vi "Circus Kaslis IPs.vi"(3 "error in (no error)":errorcluster, 4 "ID":string) -> (0 "error out":errorcluster, 1 "IP":string)   [LabVIEW 2026, in "TALOS.lvlib"]
doc: "This VI gives the IP of a PC, given its name, if it has been correctly inserted in the AEgIS_Config_Param.ini. If not present, it returns its ID (which is also its DNS name)."
uses:
  TALOS.lvlib
  Ancestor/Ancestor/Ancestor.lvclass/Ancestor.ctl
  FGV/Error Memory/Get Error Description.vi
  Get PC name.vi
  Ancestor/Ancestor/Read ID.vi
  Get Class Name.vi
  <vilib>/Utility/error.llb/Clear Errors.vi
  FGV/Error Memory/Error Memory Core.vi
  <vilib>/AdvancedString/Delimited String to 1D String Array (string).vi
  Circus Root Path.vi
  FGV/Error Memory/Error Crt Lvl checker.vi
  FGV/Error Memory/Error Memory Core.vi/40c8088d-b597-4017-91af-faa98e00292e.vi
  FGV/Error Memory/Error Memory Core.vi/d4a3ab98-063c-4e44-b43d-fbdcfe6c2be2.vi
  Global Memory.vi
  <vilib>/Utility/LVClass/Get LV Class Name.vi
  Is in Packed Library.vi
  TALOS Root path.vi
  Read CSV worksheet.vi
  Global Constants.vi
  <vilib>/Utility/error.llb/General Error Handler.vi
  Ancestor/Ancestor/Ancestor.lvclass
  <vilib>/Comparison/Equal/Equal Functor/Equal Functor.lvclass
  <vilib>/Utility/error.llb/Trim Whitespace (string).vi
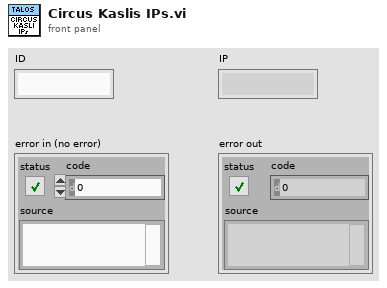
[diagram p1: front panel]
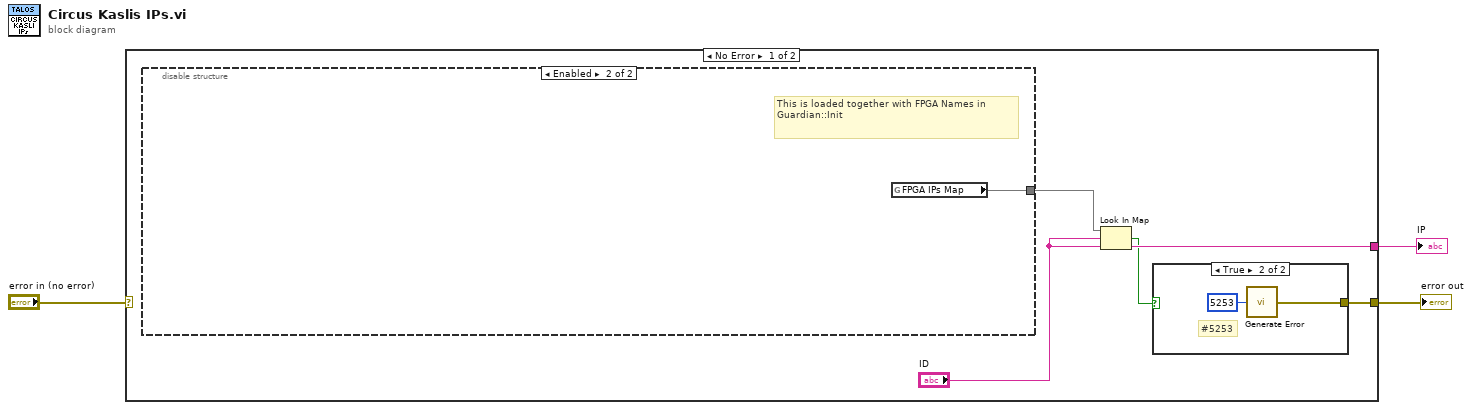
[diagram p0: block diagram]
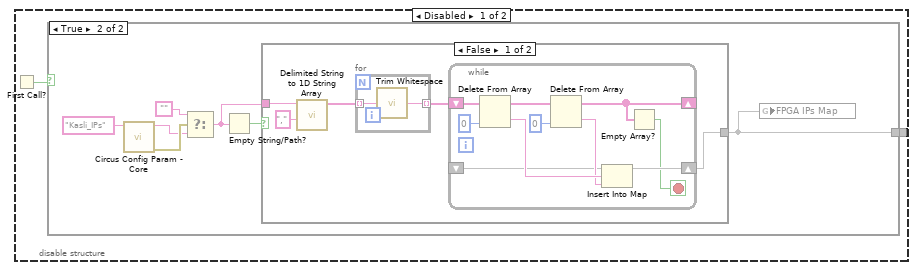
[diagram p2: hidden frame]
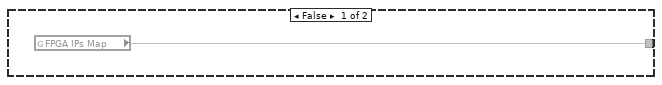
[diagram p3: hidden frame]
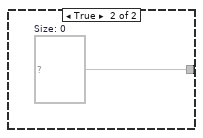
[diagram p4: hidden frame]
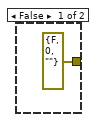
[diagram p5: hidden frame]
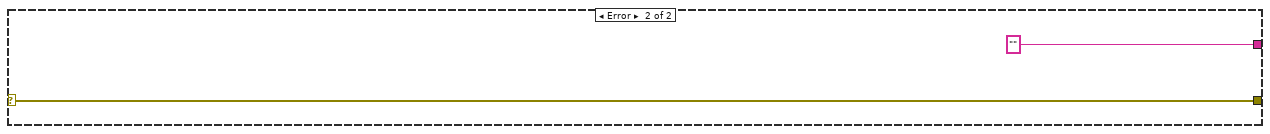
[diagram p6: hidden frame]
diagram:
  n1 = case shown="No Error" "error in (no error)" {
    selector: "error in (no error)" -> [_ w41]
    tunnel: [w6 "" ("trimmed string")] -> w3
    tunnel: [w4 w41] -> w1
    frame No Error {
      n2 = disable-structure shown="Enabled" {
        disable-tunnel: [w9 w37] -> w8
        frame Disabled {
          n3 = First Call?() -> (First Call?: T/F=w10:bool)
          n4 = case shown="True" w10 {
            tunnel: [w11 w12] -> w9
            frame False {
              n5 = global read "Global Memory.vi" "FPGA IPs Map"() -> (w11:map{string, string})
            }
            frame True {
              n6 = call "Circus Config Param - Core.vi"("Parameter Name"="Kasli_IPs") -> ("error out"=w14:errorcluster, "Output"=w13:string)  [unwired: 9 in]
              n7 = Select(t="", s=w14, f=w13) -> (s? t:f=w18:string)
              n8 = Empty String/Path?(string/path=w18) -> (empty?=w17:bool)
              n9 = case shown="False" w17 {
                tunnel: w18 -> [w22 _]
                tunnel: [w19 w36] -> w12
                frame False {
                  n10 = call-poly <vilib>:"Delimited String to 1D String Array.vi"("delimiter"=",", "delimited string"=w22) -> ("string array"=w21:string[])  [unwired: 9 in]
                  n11 = for {
                    tunnel: w21 -> [w25] mode=indexing
                    tunnel: [w24] -> w20 mode=indexing
                    n12 = call-poly <vilib>:"Trim Whitespace.vi"("string"=w25) -> ("trimmed string"=w24:string)  [unwired: 1 in]
                  }
                  n13 = while {
                    shift-right: [w29] -> w19
                    shift-left: _ -> [w28]
                    shift-right: [w27] -> _
                    shift-left: w20 -> [w35]
                    stop <- w26 stop-if-true
                    n14 = Delete From Array(array=w35, index=0) -> (deleted portion=w31:string, array with subset deleted=w32:string[])  [unwired: 1 in]
                    n15 = Delete From Array(array=w32, index=0) -> (deleted portion=w30:string, array with subset deleted=w27:string[])  [unwired: 1 in]
                    n16 = Insert Into Map(map in=w28, key=w31, value=w30) -> (map out=w29:map{string, string})  [unwired: 2 out]
                    n17 = Empty Array?(array=w27) -> (empty?=w26:bool)
                  }
                }
                frame True {
                  w36 = map{string, string} {}  # Size: 0
                }
              }
              n18 = global write "Global Memory.vi" "FPGA IPs Map"(w12) -> ()
            }
          }
        }
        frame Enabled {
          # "This is loaded together with FPGA Names in Guardian::Init"
          n19 = global read "Global Memory.vi" "FPGA IPs Map"() -> (w37:map{string, string})
        }
      }
      n20 = Look In Map(map=w8, key="ID", default value="ID") -> (key not found?=w5:bool, value=w6:string)
      n21 = case shown="True" w5 {
        tunnel: [errorcluster {"status"=FALSE, "code"=0, "source"=""} ("error out") w40] -> w4
        frame False {
        }
        frame True {
          # "#5253"
          n22 = call "Generate Error.vi"("Error Code"=5253) -> ("error out"=w40:errorcluster)  [unwired: 6 in]
        }
      }
    }
    frame Error {
    }
  }
  "IP" <- w3
  "error out" <- w1
